vi "Pre Launch Init.vi"(11 "Nested in":refnum<class "UI Template with RefNums.lvclass">) -> (0 "error out":errorcluster, 3 "Nested out":refnum<class "UI Template with RefNums.lvclass">)   [LabVIEW 2020, in "UI Template with RefNums.lvclass"]
doc: "(<B>Filename</B>: Actor Framework.lvlib:Actor.lvclass:Pre Launch Init.vi)\n\nDefines behavior that occurs after the Launch Nested Actor method is invoked but before the actor's Actor Core method begins running.\n\nBy default, this method does nothing. A descendant class may override it to define behavior."
uses:
  UI Template with RefNums.lvclass
  UI Template with RefNums.lvclass/UI Template with RefNums.ctl
  <vilib>/ActorFramework/Actor/Actor.lvclass
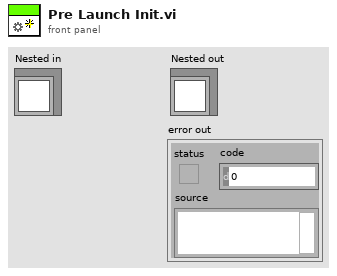
[diagram p1: front panel]
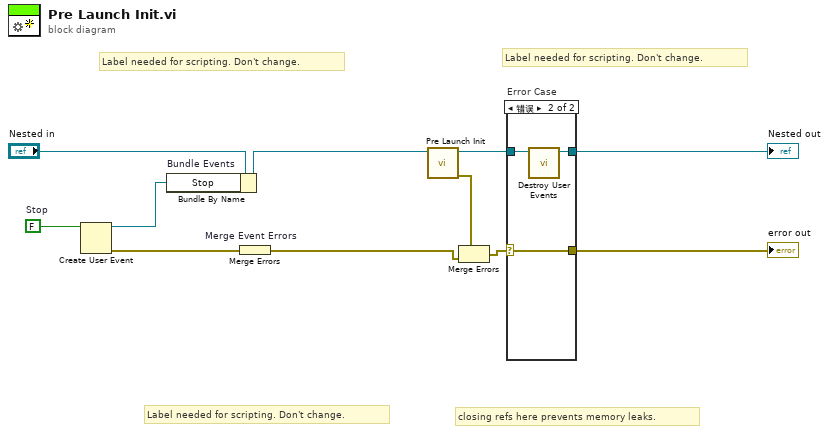
[diagram p0: block diagram]
diagram:
  w10 = FALSE  # Stop
  # "Label needed for scripting. Don't change."
  # "Label needed for scripting. Don't change."
  # "Label needed for scripting. Don't change."
  # "closing refs here prevents memory leaks."
  n1 = Create User Event(user event datatype=w10) -> (user event=w7:refnum<user-event>, error out=w9:errorcluster)  [unwired: 1 in]
  n2 = Bundle By Name "Bundle Events"(cluster="Nested in", "Stop"=w7) -> (w4:refnum<class "UI Template with RefNums.lvclass">)
  n3 = Merge Errors "Merge Event Errors"(w9) -> (w1:errorcluster)
  n4 = call-parent "Pre Launch Init.vi"("Actor in"=w4) -> ("error out"=w3:errorcluster, "Actor out"=w5:refnum<class "UI Template with RefNums.lvclass">)  [unwired: 9 in]
  n5 = Merge Errors(w3, w1) -> (w2:errorcluster)
  n6 = case "Error Case" shown="错误" w2 {
    selector: w2 -> [w12 w16]
    tunnel: w5 -> [w13 w15]
    tunnel: [w13 w14] -> w8
    tunnel: [w12 w16] -> w6
    frame No Error {
    }
    frame Error {
      n7 = call "Destroy User Events.vi"("UI Template in"=w15) -> ("UI Template out"=w14:refnum<class "UI Template with RefNums.lvclass">)  [unwired: 10 in]
    }
  }
  "error out" <- w6
  "Nested out" <- w8
